vi "Process_Meas_Data.vi"(4 "All queue elements?":bool, 6 "Queues":T4, 7 "One Seconds in":T1 {"Slave"."Ch1 High" format="%0.0f"; "Master"."Ch1 High" format="%0.0f"}, 8 "Status/Errors in":refnum<vi>, 10 "Process data parameters in":T5={"Stop loop"={"Settings changed?"=FALSE, "Stop?"=refnum}, "Button refs"={"Stop program"=refnum, "Save settings"=refnum, "DAQ mode"=refnum, "Reset settings"=refnum, "Apply settings"=refnum, "Reset MAS"=refnum, "Reset SLV"=refnum, "Local DBase?"=refnum, "Last value DBase"=FALSE, "Database"=refnum, "Calibration"=refnum, "Save settings 2"=refnum}, "Process messages"={"Process message mode"=enum."Error", "Slave data?"=FALSE, "Length get settings message"=0, "Delta time"=0.0, "Data_Filter"={"Filter_Data"=FALSE, "Use_Thresh"=FALSE, "Reduce data?"=FALSE}, "Time_difference_stack"=[], "Starting sec"=0, "Ending sec"=0, "Ending sec 2"=0, "MAS_Page_Thresh"=refnum, "SLV_Page_Thresh"=refnum, "Database"=refnum}, "Settings state"={"MAS locked?"=refnum, "SLV locked?"=refnum}, "Mode"={"Mode"=enum."Dialog", "Expert?"=FALSE, "Dialog?"=FALSE}, "Alignment parameters"=refnum, "Timer parameters"=refnum, "Files"={"Path config file"=path "", "Path def. ini file"=path "", "Path ini file 1"=path "", "Path ini file 2"=path "", "Path RBF file"=path ""}, "Time difference"=refnum, "Alignment"={"GEN_Page_Calibrate"=refnum, "MAS_Page_Gain"=refnum, "MAS_Page_Offset"=refnum, "SLV_Page_Gain"=refnum, "SLV_Page_Offset"=refnum, "MAS_Page_Common"=refnum, "SLV_Page_Common"=refnum}, "Page Statistics"=refnum}, 11 "Devices in":T14) -> (0 "Status/Errors out":refnum<vi>, 2 "Process data parameters out":T5={"Stop loop"={"Settings changed?"=FALSE, "Stop?"=refnum}, "Button refs"={"Stop program"=refnum, "Save settings"=refnum, "DAQ mode"=refnum, "Reset settings"=refnum, "Apply settings"=refnum, "Reset MAS"=refnum, "Reset SLV"=refnum, "Local DBase?"=refnum, "Last value DBase"=FALSE, "Database"=refnum, "Calibration"=refnum, "Save settings 2"=refnum}, "Process messages"={"Process message mode"=enum."Error", "Slave data?"=FALSE, "Length get settings message"=0, "Delta time"=0.0, "Data_Filter"={"Filter_Data"=FALSE, "Use_Thresh"=FALSE, "Reduce data?"=FALSE}, "Time_difference_stack"=[], "Starting sec"=0, "Ending sec"=0, "Ending sec 2"=0, "MAS_Page_Thresh"=refnum, "SLV_Page_Thresh"=refnum, "Database"=refnum}, "Settings state"={"MAS locked?"=refnum, "SLV locked?"=refnum}, "Mode"={"Mode"=enum."Dialog", "Expert?"=FALSE, "Dialog?"=FALSE}, "Alignment parameters"=refnum, "Timer parameters"=refnum, "Files"={"Path config file"=path "", "Path def. ini file"=path "", "Path ini file 1"=path "", "Path ini file 2"=path "", "Path RBF file"=path ""}, "Time difference"=refnum, "Alignment"={"GEN_Page_Calibrate"=refnum, "MAS_Page_Gain"=refnum, "MAS_Page_Offset"=refnum, "SLV_Page_Gain"=refnum, "SLV_Page_Offset"=refnum, "MAS_Page_Common"=refnum, "SLV_Page_Common"=refnum}, "Page Statistics"=refnum}, 3 "Devices out":T14, 5 "One Seconds out":T1 {"Slave"."Ch1 High" format="%0.0f"; "Master"."Ch1 High" format="%0.0f"})   [LabVIEW 2013]
uses:
  Controls/Devices.ctl
  Controls/Process_Data_Parameters.ctl
  Controls/Stop_Loop.ctl
  Controls/Button_Refs.ctl
  Controls/Process_Messages.ctl
  Controls/Process_Message_Mode.ctl
  Controls/Settings_State.ctl
  Controls/Mode.ctl
  Controls/Files.ctl
  Controls/Page_Calibration.ctl
  Controls/Queues.ctl
  Controls/One_Second.ctl
  Controls/GPS_Timestamp.ctl
  Controls/One_Seconds.ctl
  Controls/Found_SLV_Data.ctl
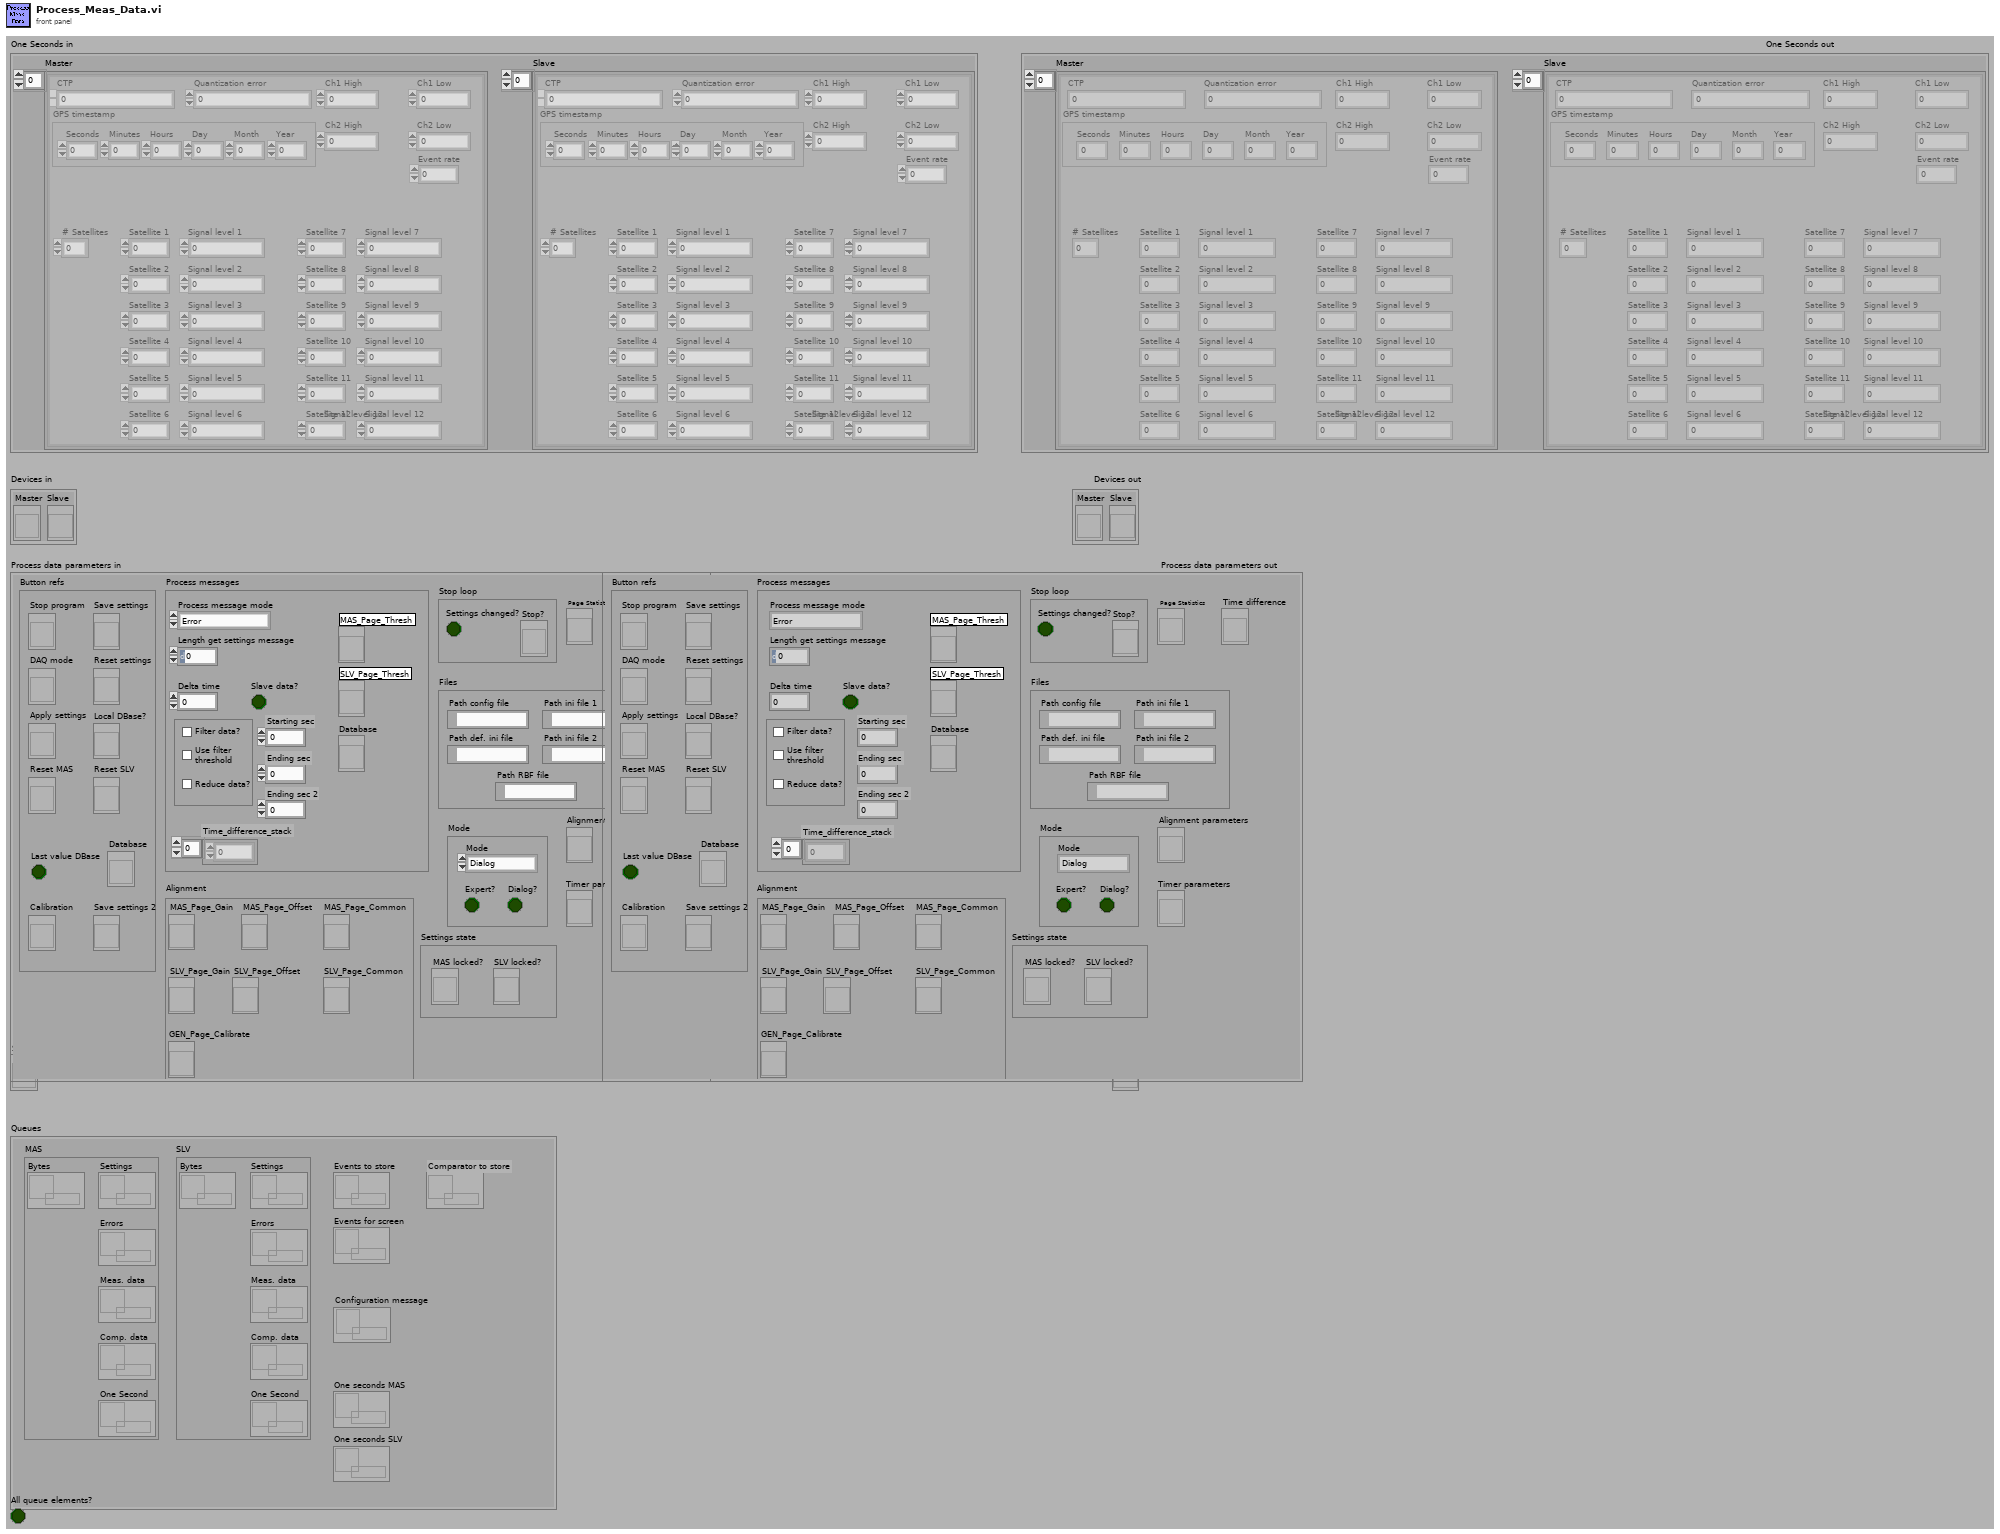
[diagram p1: front panel]
types:
  T1 = typedef "One_Seconds.ctl" = cluster{"Master":T2[], "Slave":T2[]}
  T2 = typedef "One_Second.ctl" = cluster{"GPS timestamp":T3, "CTP":u32, "Quantization error":u32, "Ch1 High":u16, "Ch1 Low":u16, "Ch2 High":u16, "Ch2 Low":u16, "Event rate":u16, "# Satellites":u8, "Satellite 1":u8, "Satellite 2":u8, "Satellite 3":u8, "Satellite 4":u8, "Satellite 5":u8, "Satellite 6":u8, "Signal level 1":sgl, "Signal level 2":sgl, "Signal level 3":sgl, "Signal level 4":sgl, "Signal level 5":sgl, "Signal level 6":sgl, "Satellite 7":u8, "Satellite 8":u8, "Satellite 9":u8, "Satellite 10":u8, "Satellite 11":u8, "Satellite 12":u8, "Signal level 7":sgl, "Signal level 8":sgl, "Signal level 9":sgl, "Signal level 10":sgl, "Signal level 11":sgl, "Signal level 12":sgl}
  T3 = typedef "GPS_Timestamp.ctl" = cluster{"Seconds":u8, "Minutes":u8, "Hours":u8, "Day":u8, "Month":u8, "Year":u16}
  T4 = typedef "Queues.ctl" = cluster{"MAS":cluster{"Bytes":refnum<queue>, "Settings":refnum<queue>, "Errors":refnum<queue>, "Meas. data":refnum<queue>, "One Second":refnum<queue>, "Comp. data":refnum<queue>}, "SLV":cluster{"Bytes":refnum<queue>, "Settings":refnum<queue>, "Errors":refnum<queue>, "Meas. data":refnum<queue>, "One Second":refnum<queue>, "Comp. data":refnum<queue>}, "Events to store":refnum<queue>, "Events for screen":refnum<queue>, "One seconds MAS":refnum<queue>, "One seconds SLV":refnum<queue>, "Configuration message":refnum<queue>, "Comparator to store":refnum<queue>}
  T5 = typedef "Process_Data_Parameters.ctl" = cluster{"Stop loop":T6, "Button refs":T7, "Process messages":T8, "Settings state":T10, "Mode":T11, "Alignment parameters":refnum<vi>, "Timer parameters":refnum<vi>, "Files":T12, "Time difference":refnum<vi>, "Alignment":T13, "Page Statistics":refnum<vi>}
  T6 = typedef "Stop_Loop.ctl" = cluster{"Settings changed?":bool, "Stop?":refnum<vi>}
  T7 = typedef "Button_Refs.ctl" = cluster{"Stop program":refnum<vi>, "Save settings":refnum<vi>, "DAQ mode":refnum<vi>, "Reset settings":refnum<vi>, "Apply settings":refnum<vi>, "Reset MAS":refnum<vi>, "Reset SLV":refnum<vi>, "Local DBase?":refnum<vi>, "Last value DBase":bool, "Database":refnum<vi>, "Calibration":refnum<vi>, "Save settings 2":refnum<vi>}
  T8 = typedef "Process_Messages.ctl" = cluster{"Process message mode":T9, "Slave data?":bool, "Length get settings message":i32, "Delta time":dbl, "Data_Filter":cluster{"Filter_Data":bool, "Use_Thresh":bool, "Reduce data?":bool}, "Time_difference_stack":u64[], "Starting sec":u64, "Ending sec":u64, "Ending sec 2":u64, "MAS_Page_Thresh":refnum<vi>, "SLV_Page_Thresh":refnum<vi>, "Database":refnum<vi>}
  T9 = typedef "Process_Message_Mode.ctl" = enum16{"Error", "Measurement data", "Comparator data", "One Second"}
  T10 = typedef "Settings_State.ctl" = cluster{"MAS locked?":refnum<vi>, "SLV locked?":refnum<vi>}
  T11 = typedef "Mode.ctl" = cluster{"Mode":enum8{"Stop", "Dialog", "Hisparc II", "Hisparc II DAQ", "Alignment"}, "Expert?":bool, "Dialog?":bool}
  T12 = typedef "Files.ctl" = cluster{"Path config file":path, "Path def. ini file":path, "Path ini file 1":path, "Path ini file 2":path, "Path RBF file":path}
  T13 = typedef "Page_Calibration.ctl" = cluster{"GEN_Page_Calibrate":refnum<vi>, "MAS_Page_Gain":refnum<vi>, "MAS_Page_Offset":refnum<vi>, "SLV_Page_Gain":refnum<vi>, "SLV_Page_Offset":refnum<vi>, "MAS_Page_Common":refnum<vi>, "SLV_Page_Common":refnum<vi>}
  T14 = typedef "Devices.ctl" = cluster{"Master":refnum<vi>, "Slave":refnum<vi>}
  T15 = enum8{"Stop", "Dialog", "Hisparc II", "Hisparc II DAQ", "Alignment"}
  T16 = typedef "Found_SLV_Data.ctl" = cluster{"Found SLV data?":bool, "Wait for SLV data?":bool}
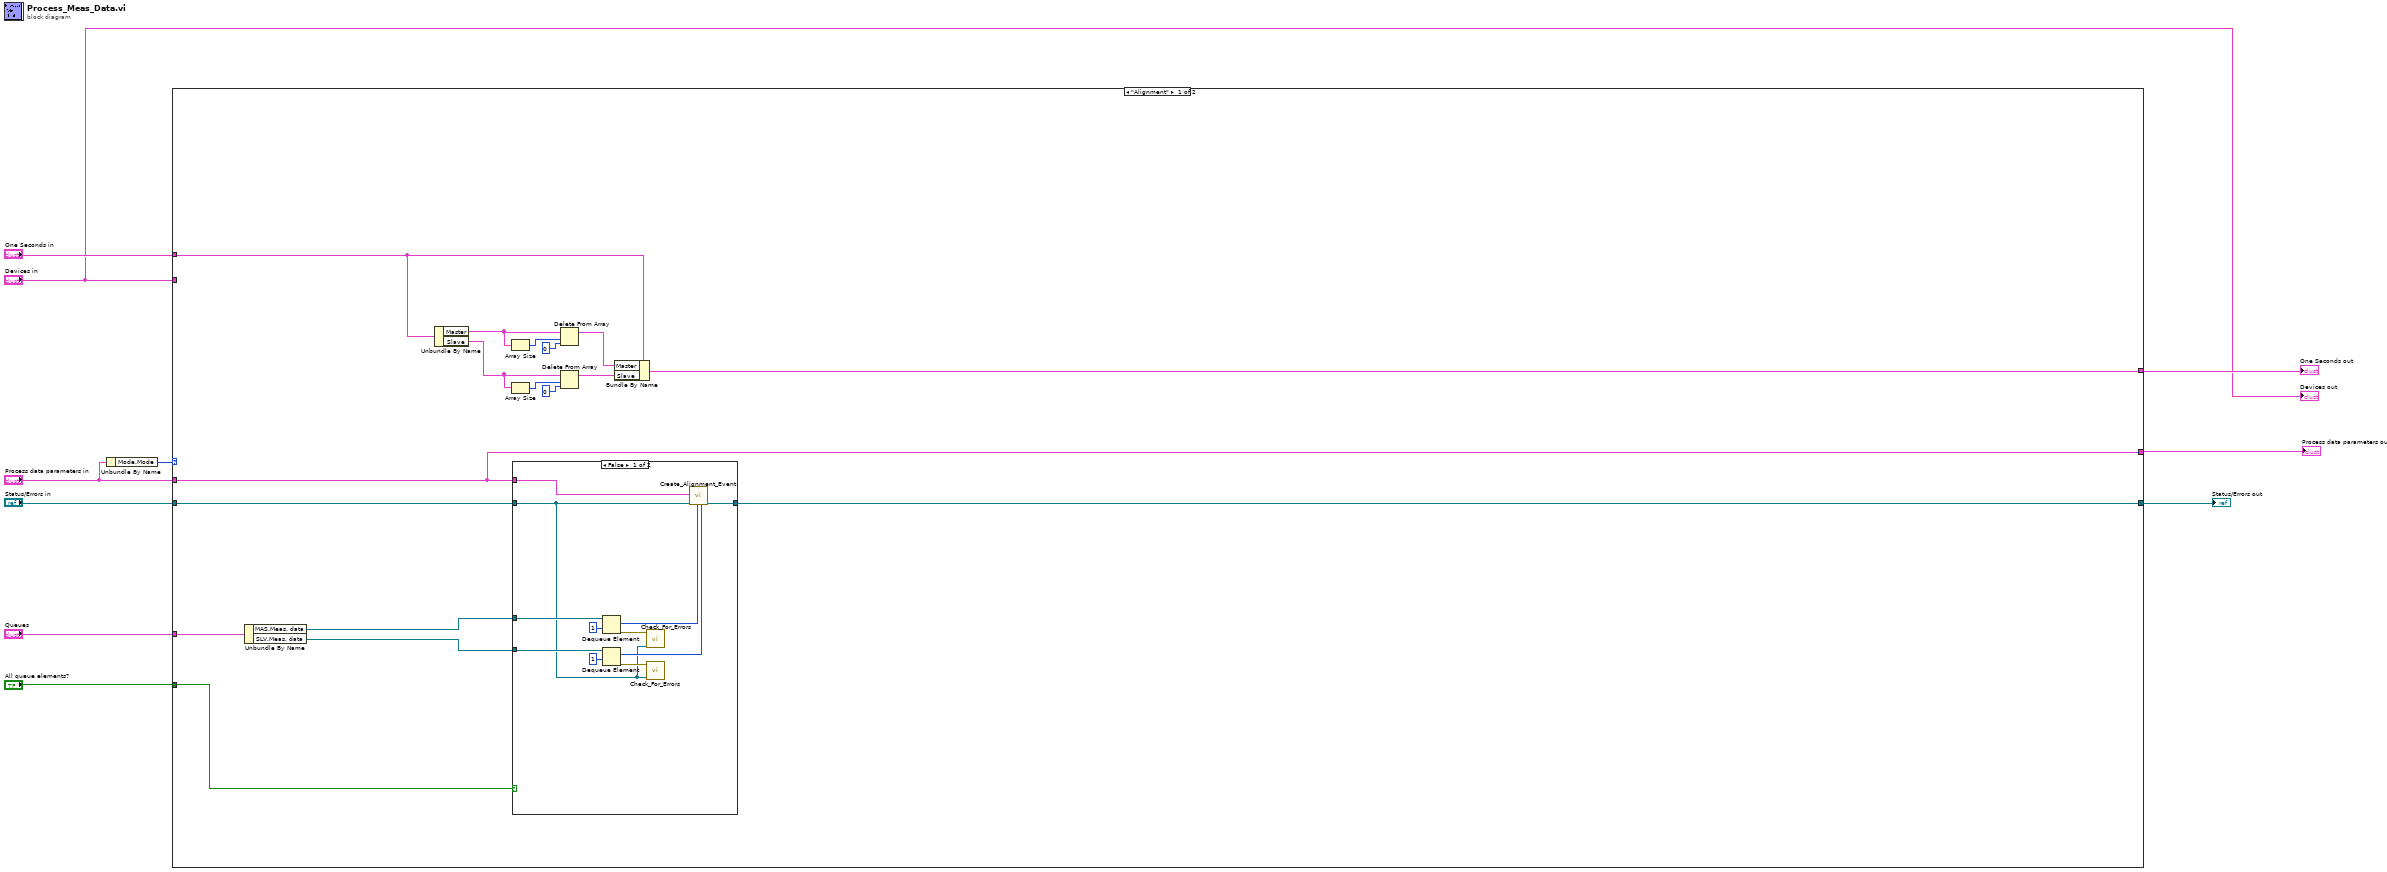
[diagram p0: block diagram]
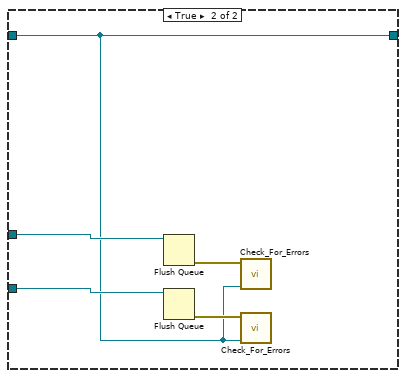
[diagram p2: hidden frame]
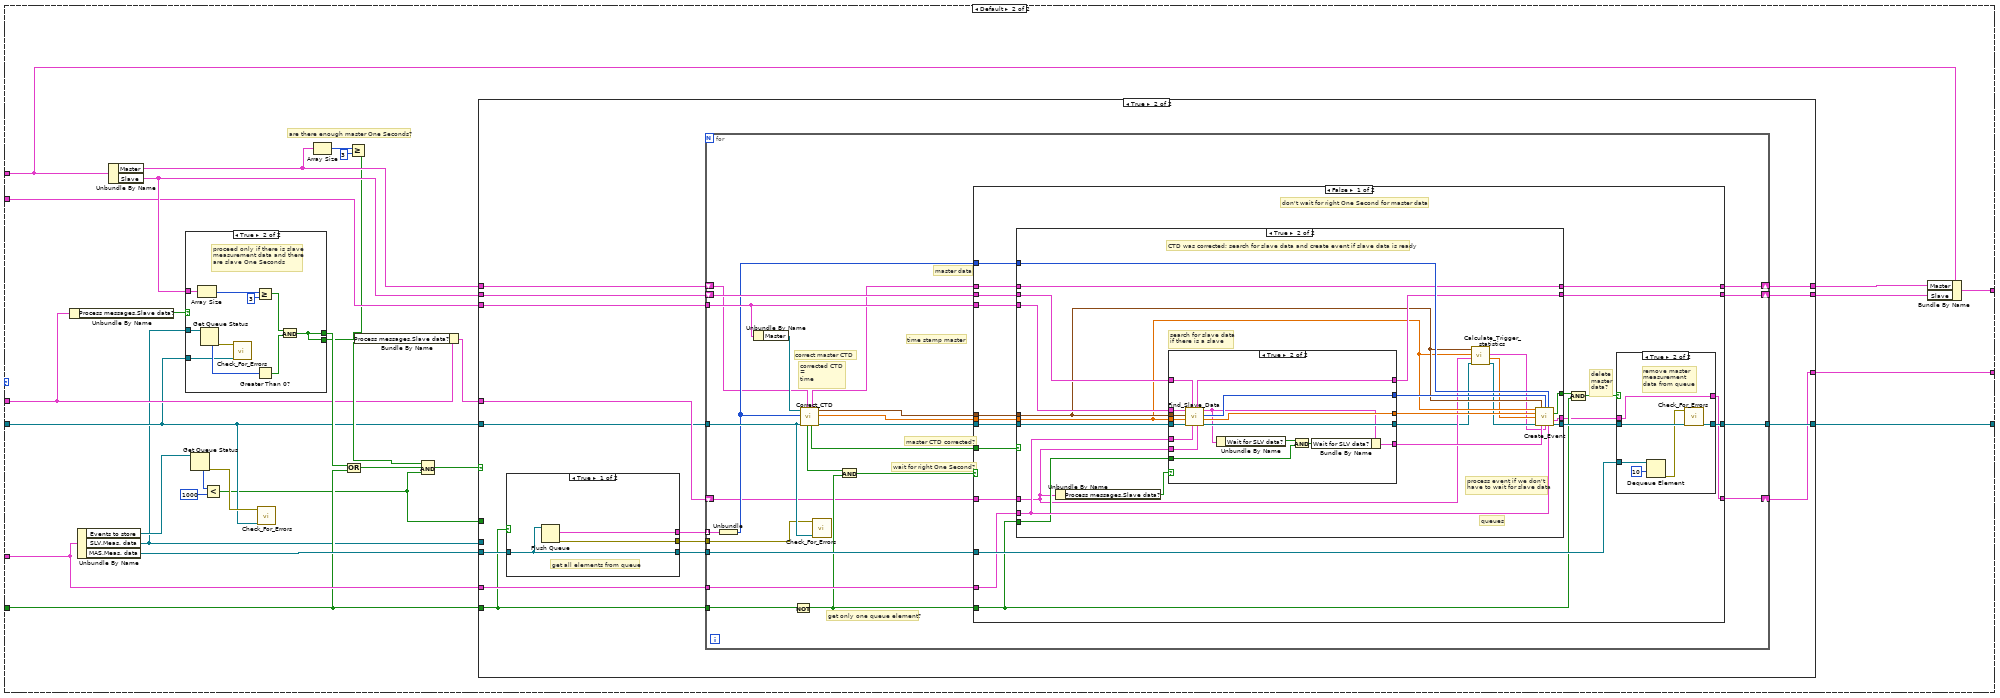
[diagram p3: hidden frame]
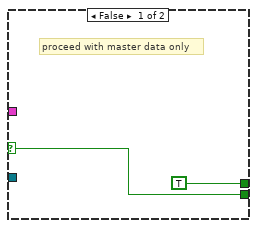
[diagram p4: hidden frame]
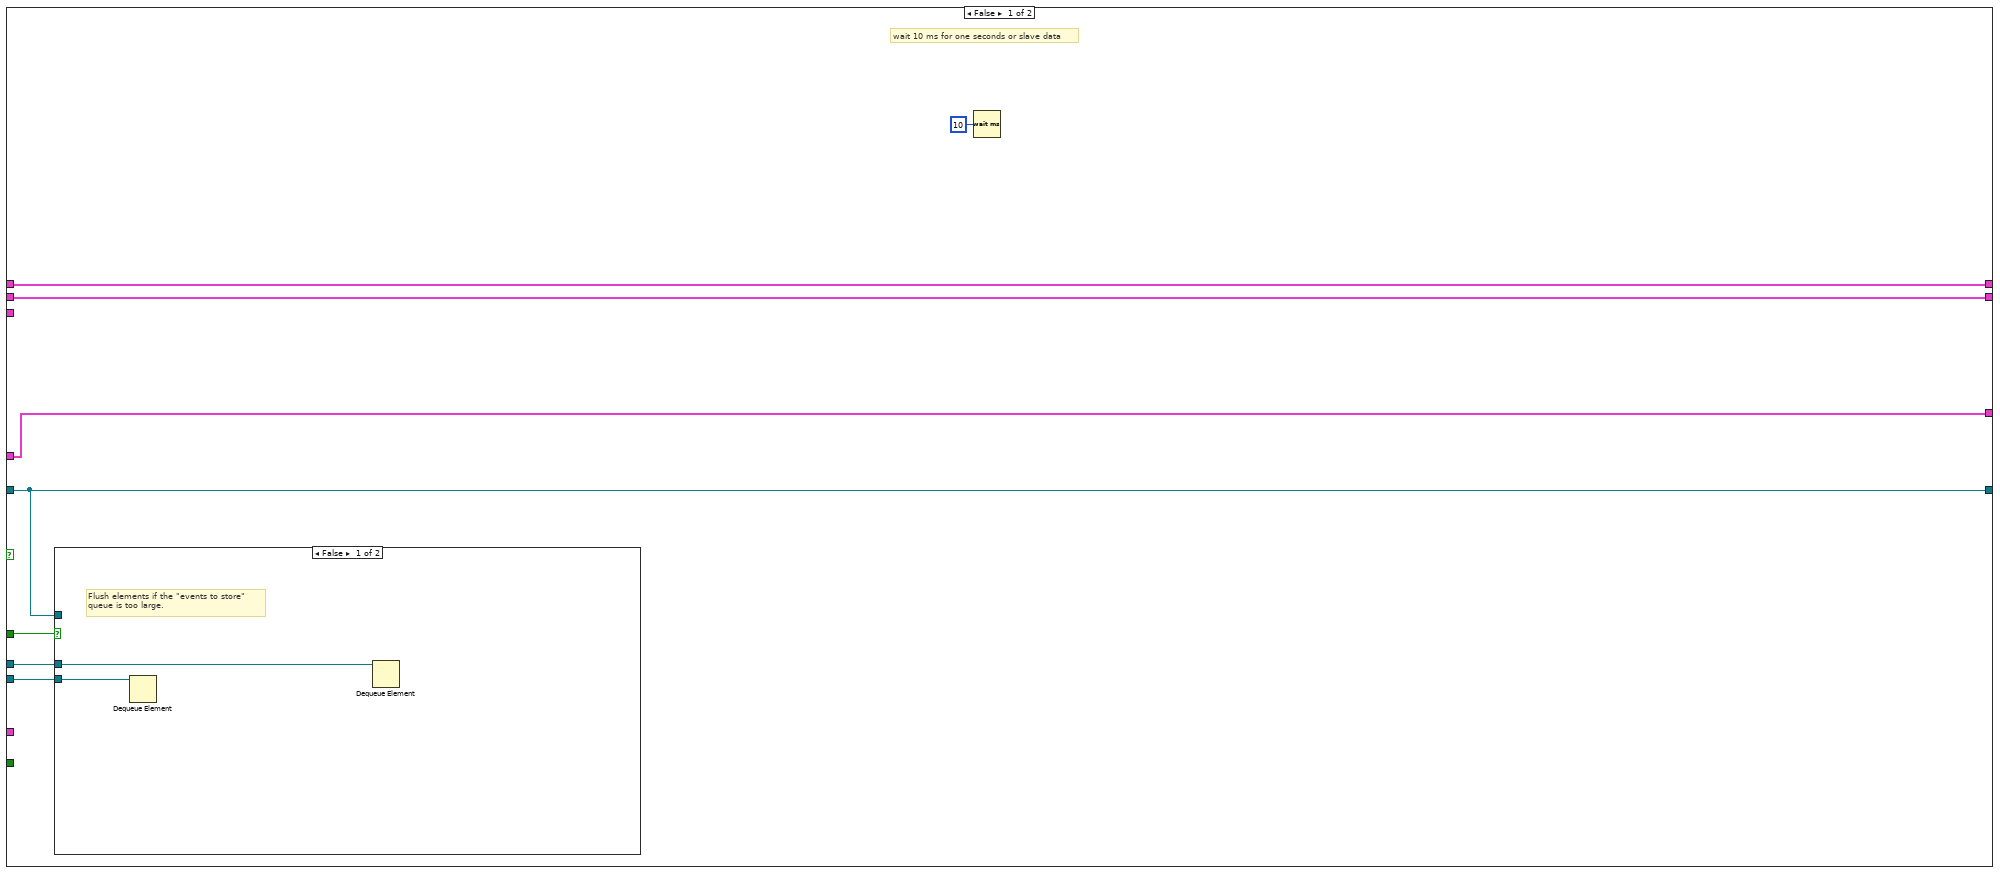
[diagram p5: hidden frame]
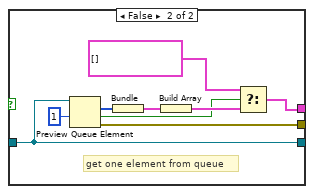
[diagram p7: hidden frame]
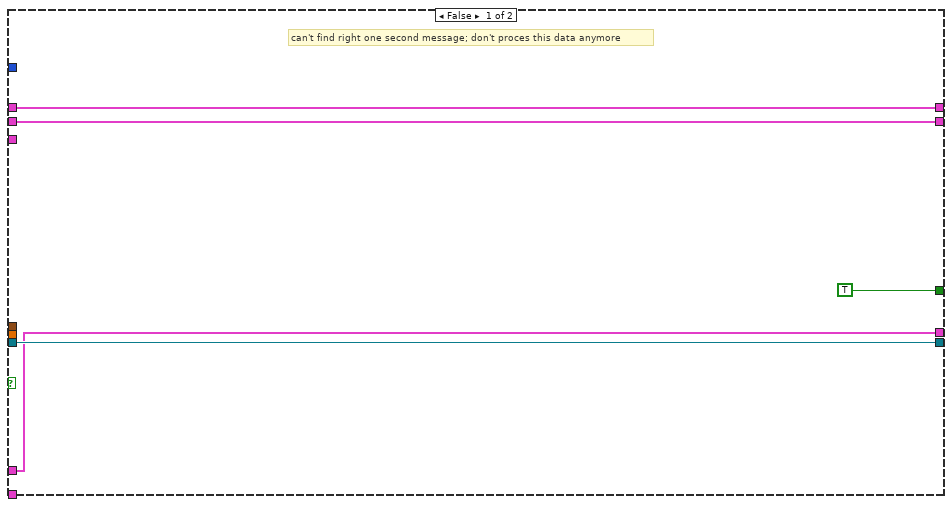
[diagram p9: hidden frame]
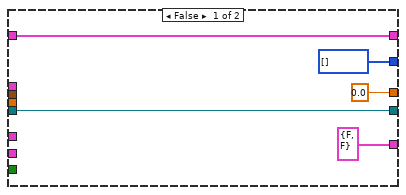
[diagram p10: hidden frame]
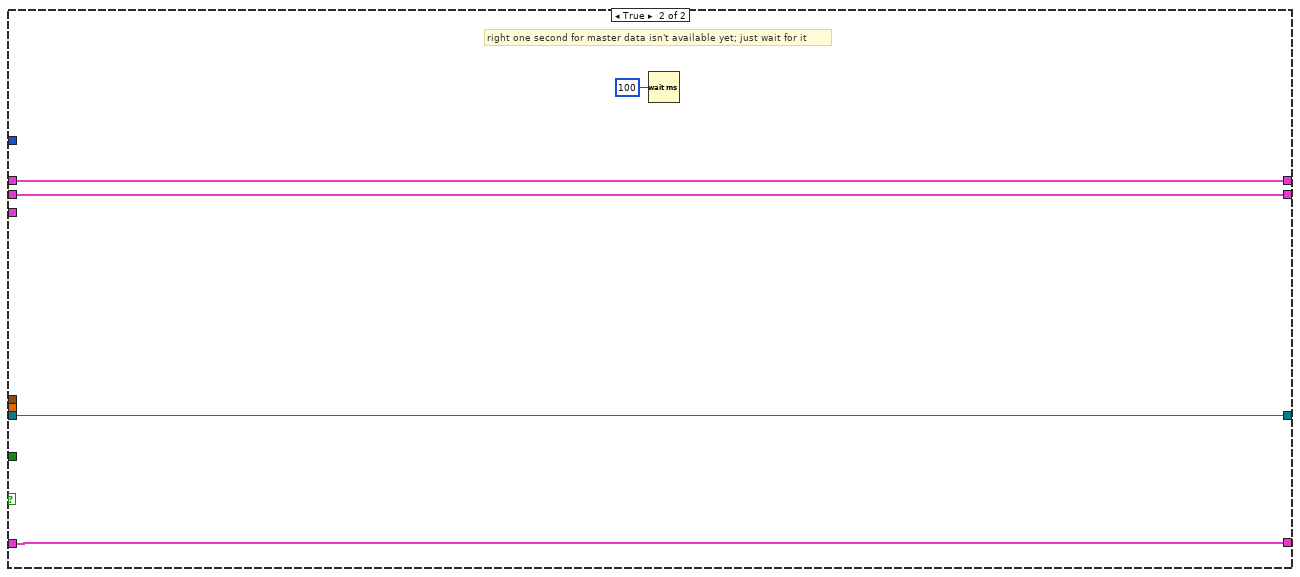
[diagram p11: hidden frame]
diagram:
  n1 = Unbundle By Name("Process data parameters in") -> ("Mode.Mode"=w5:T15)
  n2 = case shown="\"Alignment\"" w5 {
    tunnel: [w22 w72] -> w3
    tunnel: [w12 w68] -> w10
    tunnel: "One Seconds in" -> [w13 w67]
    tunnel: "Queues" -> [w27 w65]
    tunnel: "All queue elements?" -> [w26 w61]
    tunnel: "Devices in" -> [_ w59]
    tunnel: "Status/Errors in" -> [w25 w47]
    tunnel: "Process data parameters in" -> [w11 w52]
    tunnel: [w11 w44] -> w1
    frame "Alignment" {
      n3 = Unbundle By Name(w27) -> ("MAS.Meas. data"=w24:refnum<queue>, "SLV.Meas. data"=w23:refnum<queue>)
      n4 = Unbundle By Name(w13) -> ("Master"=w21:T2[], "Slave"=w16:T2[])
      n5 = Array Size(array=w21) -> (size(s)=w20:i32)
      n6 = Array Size(array=w16) -> (size(s)=w18:i32)
      n7 = case shown="False" w26 {
        tunnel: w25 -> [w30 w39]
        tunnel: w24 -> [w38 w41]
        tunnel: w23 -> [w35 w40]
        tunnel: w11 -> [w29 _]
        tunnel: [w28 w39] -> w22
        frame False {
          n8 = Dequeue Element(queue=w38, timeout in ms (-1)=1) -> (element=w34:u8[], error out=w32:errorcluster)  [unwired: 1 in, 2 out]
          n9 = Dequeue Element(queue=w35, timeout in ms (-1)=1) -> (element=w33:u8[], error out=w31:errorcluster)  [unwired: 1 in, 2 out]
          n10 = call "Check_For_Errors.vi"("Status/Errors in"=w30, "error in"=w32) -> ()  [unwired: 10 out]
          n11 = call "Check_For_Errors.vi"("Status/Errors in"=w30, "error in"=w31) -> ()  [unwired: 10 out]
          n12 = call "Create_Alignment_Event.vi"("Slave data"=w33, "Master data"=w34, "Status/Errors in"=w30, "Process data parameters in"=w29) -> ("Status/Errors out"=w28:refnum<vi>)  [unwired: 2 in, 5 out]
        }
        frame True {
          n13 = Flush Queue(queue=w41) -> (error out=w43:errorcluster)  [unwired: 1 in, 2 out]
          n14 = Flush Queue(queue=w40) -> (error out=w42:errorcluster)  [unwired: 1 in, 2 out]
          n15 = call "Check_For_Errors.vi"("Status/Errors in"=w39, "error in"=w43) -> ()  [unwired: 10 out]
          n16 = call "Check_For_Errors.vi"("Status/Errors in"=w39, "error in"=w42) -> ()  [unwired: 10 out]
        }
      }
      n17 = Delete From Array(array=w21, length=w20, index=0) -> (array with subset deleted=w15:T2[])  [unwired: 1 out]
      n18 = Delete From Array(array=w16, length=w18, index=0) -> (array with subset deleted=w14:T2[])  [unwired: 1 out]
      n19 = Bundle By Name(cluster=w13, "Master"=w15, "Slave"=w14) -> (w12:T1)
    }
    frame Default {
      # "are there enough master One Seconds?"
      n20 = Unbundle By Name(w52) -> ("Process messages.Slave data?"=w71:bool)
      n21 = Unbundle By Name(w65) -> ("Events to store"=w51:refnum<queue>, "SLV.Meas. data"=w46:refnum<queue>, "MAS.Meas. data"=w66:refnum<queue>)
      n22 = Unbundle By Name(w67) -> ("Master"=w56:T2[], "Slave"=w60:T2[])
      n23 = case shown="True" w71 {
        selector: w71 -> [w73 _]
        tunnel: [TRUE w77] -> w63
        tunnel: w46 -> [_ w82]
        tunnel: w47 -> [_ w81]
        tunnel: w60 -> [_ w80]
        tunnel: [w73 w77] -> w62
        frame False {
          # "proceed with master data only"
        }
        frame True {
          # "proceed only if there is slave\nmeasurement data and there\nare slave One Seconds"
          n24 = Array Size(array=w80) -> (size(s)=w76:i32)
          n25 = Get Queue Status(queue=w82) -> (error out=w83:errorcluster, # elements in queue=w84:i32)  [unwired: 1 in, 7 out]
          n26 = call "Check_For_Errors.vi"("Status/Errors in"=w81, "error in"=w83) -> ()  [unwired: 10 out]
          n27 = Greater Or Equal?(x=w76, y=3) -> (x >= y?=w78:bool)
          n28 = Greater Than 0?(x=w84) -> (x > 0?=w79:bool)
          n29 = And(x=w78, y=w79) -> (x .and. y?=w77:bool)
        }
      }
      n30 = Get Queue Status(queue=w51) -> (error out=w48:errorcluster, # elements in queue=w49:i32)  [unwired: 1 in, 7 out]
      n31 = Less?(x=w49, y=1000) -> (x < y?=w45:bool)
      n32 = call "Check_For_Errors.vi"("Status/Errors in"=w47, "error in"=w48) -> ()  [unwired: 10 out]
      n33 = Array Size(array=w56) -> (size(s)=w58:i32)
      n34 = Or(x=w63, y=w61) -> (x .or. y?=w54:bool)
      n35 = Greater Or Equal?(x=w58, y=3) -> (x >= y?=w53:bool)
      n36 = Bundle By Name(cluster=w52, "Process messages.Slave data?"=w62) -> (w64:T5)
      n37 = Compound Arithmetic op=AND(w53, w54, w45) -> (w55:bool)
      n38 = case shown="True" w55 {
        tunnel: [w87 w109] -> w72
        tunnel: w64 -> [w85 w108]
        tunnel: w47 -> [w87 w107]
        tunnel: w66 -> [w89 w105]
        tunnel: w59 -> [_ w104]
        tunnel: w56 -> [w90 w100]
        tunnel: [w90 w103] -> w70
        tunnel: w60 -> [w91 w102]
        tunnel: [w91 w99] -> w69
        tunnel: w65 -> [_ w101]
        tunnel: w61 -> [_ w96]
        tunnel: w46 -> [w88 _]
        tunnel: w45 -> [w86 _]
        tunnel: [w85 w95] -> w44
        frame False {
          # "wait 10 ms for one seconds or slave data"
          n39 = case shown="False" w86 {
            tunnel: w89 -> [w94 _]
            tunnel: w88 -> [w93 _]
            tunnel: w87 -> [_ _]
            frame False {
              # "Flush elements if the \"events to store\" \nqueue is too large."
              n40 = Dequeue Element(queue=w94) -> ()  [unwired: 1 in, 5 out]
              n41 = Dequeue Element(queue=w93) -> ()  [unwired: 1 in, 5 out]
            }
            frame True {
            }
          }
          n42 = Wait (ms)(milliseconds to wait=u32 10) -> ()  [unwired: 1 out]
        }
        frame True {
          n43 = case shown="True" w96 {
            tunnel: [w112 w121] -> w106
            tunnel: w105 -> [w110 w118]
            tunnel: [w111 w114] -> w98
            tunnel: [w110 w118] -> w97
            frame True {
              # "get all elements from queue"
              n44 = Flush Queue(queue=w110) -> (remaining elements=w111:cluster{u8[]}[], error out=w112:errorcluster)  [unwired: 1 in, 1 out]
            }
            frame False {
              # "get one element from queue"
              n45 = Preview Queue Element(queue=w118, timeout in ms (-1)=1) -> (element=w120:u8[], timed out?=w115:bool, error out=w121:errorcluster)  [unwired: 1 in, 1 out]
              n46 = Bundle(w120) -> (w119:cluster{u8[]})  [unwired: 1 in]
              n47 = Build Array(w119) -> (w116:cluster{u8[]}[])
              n48 = Select(t=cluster{u8[]}[] [], s=w115, f=w116) -> (s? t:f=w114:cluster{u8[]}[])
            }
          }
          n49 = for {
            tunnel: [w144] -> w109
            tunnel: w107 -> [w143]
            tunnel: w106 -> [w142]
            tunnel: w97 -> [w141]
            tunnel: w98 -> [w140] mode=indexing
            tunnel: w104 -> [w139]
            tunnel: w101 -> [w138]
            shift-right: [w126] -> w103
            shift-left: w100 -> [w131]
            shift-right: [w136] -> w99
            shift-left: w102 -> [w137]
            tunnel: w96 -> [w134]
            shift-right: [w128] -> w95
            shift-left: w108 -> [w122]
            # "get only one queue element?"
            # "time stamp master"
            # "corrected CTD\n=\ntime"
            # "master data"
            # "correct master CTD"
            # "master CTD corrected?"
            # "wait for right One Second?"
            n50 = Unbundle(w140) -> (w135:u8[])
            n51 = Unbundle By Name(w139) -> ("Master"=w145:refnum<vi>)
            n52 = Not(x=w134) -> (.not. x?=w132:bool)
            n53 = call "Correct_CTD.vi"("One Second in"=w131, "Status/Errors in"=w143, "Message in"=w135, "Device in"=w145) -> ("Status/Errors out"=w123:refnum<vi>, "Time"=w125:dbl, "GPS timestamp out"=w124:T3, "CTD corrected?"=w129:bool, "One Second out"=w127:T2[], "Wait for tick count?"=w130:bool)  [unwired: 2 out]
            n54 = call "Check_For_Errors.vi"("Status/Errors in"=w143, "error in"=w142) -> ()  [unwired: 10 out]
            n55 = And(x=w130, y=w132) -> (x .and. y?=w133:bool)
            n56 = case shown="False" w133 {
              tunnel: [w156 w226] -> w144
              tunnel: w123 -> [w165 w226]
              tunnel: w139 -> [w164 _]
              tunnel: w129 -> [w162 _]
              tunnel: w141 -> [w163 _]
              tunnel: w122 -> [w158 w223]
              tunnel: w124 -> [w160 _]
              tunnel: w125 -> [w159 _]
              tunnel: w135 -> [w161 _]
              tunnel: w137 -> [w155 w224]
              tunnel: [w154 w224] -> w136
              tunnel: w138 -> [w153 _]
              tunnel: w132 -> [w150 _]
              tunnel: [w148 w223] -> w128
              tunnel: w127 -> [w147 w222]
              tunnel: [w146 w222] -> w126
              frame False {
                # "delete\nmaster\ndata?"
                # "don't wait for right One Second for master data"
                n57 = case shown="True" w162 {
                  tunnel: w164 -> [_ w199]
                  tunnel: [w178 w190] -> w157
                  tunnel: w165 -> [w178 w200]
                  tunnel: w160 -> [_ w185]
                  tunnel: w159 -> [_ w184]
                  tunnel: [TRUE w192] -> w151
                  tunnel: w161 -> [_ w196]
                  tunnel: w158 -> [w175 w183]
                  tunnel: w155 -> [w176 w197]
                  tunnel: [w176 w187] -> w154
                  tunnel: w153 -> [_ w193]
                  tunnel: w150 -> [_ w191]
                  tunnel: [w175 w188] -> w149
                  tunnel: w147 -> [w174 w186]
                  tunnel: [w174 w186] -> w146
                  frame False {
                    # "can't find right one second message; don't proces this data anymore"
                  }
                  frame True {
                    # "search for slave data\nif there is a slave"
                    # "process event if we don't\nhave to wait for slave data"
                    # "queues"
                    # "CTD was corrected; search for slave data and create event if slave data is ready"
                    n58 = Unbundle By Name(w183) -> ("Process messages.Slave data?"=w198:bool)
                    n59 = case shown="True" w198 {
                      tunnel: w200 -> [w205 w213]
                      tunnel: [w205 w211] -> w182
                      tunnel: w199 -> [_ w221]
                      tunnel: w185 -> [_ w220]
                      tunnel: w184 -> [_ w219]
                      tunnel: [u8[] [] ("Slave data") w218] -> w195
                      tunnel: [0.0 ("CTDM slave") w217] -> w194
                      tunnel: w197 -> [w202 w216]
                      tunnel: [w202 w215] -> w187
                      tunnel: w193 -> [_ w214]
                      tunnel: w183 -> [_ w212]
                      tunnel: [T16 {"Found SLV data?"=FALSE, "Wait for SLV data?"=FALSE} ("Found SLV data?") w206] -> w189
                      tunnel: w191 -> [_ w209]
                      frame False {
                      }
                      frame True {
                        n60 = call "Find_Slave_Data.vi"("Process data parameters in"=w212, "Queues"=w214, "One Second in"=w216, "Status/Errors in"=w213, "Time master"=w219, "GPS timestamp master"=w220, "Devices"=w221) -> ("Status/Errors out"=w211:refnum<vi>, "Time delta slave"=w217:dbl, "Slave data"=w218:u8[], "Found SLV data?"=w208:T16, "One Second out"=w215:T2[])
                        n61 = Unbundle By Name(w208) -> ("Wait for SLV data?"=w210:bool)
                        n62 = And(x=w210, y=w209) -> (x .and. y?=w207:bool)
                        n63 = Bundle By Name(cluster=w208, "Wait for SLV data?"=w207) -> (w206:T16)
                      }
                    }
                    n64 = call "Calculate_Trigger_statistics.vi"("Status/Errors in"=w182, "Process data parameters in"=w183, "Time"=w184, "GPS timestamp in"=w185) -> ("Status/Errors out"=w181:refnum<vi>, "Trigger rate /s"=w180:dbl, "Process data parameters out"=w179:T5)  [unwired: 5 out]
                    n65 = call "Create_Event.vi"("Time master"=w184, "GPS timestamp master"=w185, "Slave data"=w195, "Master data"=w196, "Time delta slave"=w194, "Trigger rate /m"=w180, "Status/Errors in"=w181, "Found SLV data?"=w189, "Process data parameters in"=w179, "Queues"=w193) -> ("Delete master data?"=w192:bool, "Process data parameters out"=w188:T5, "Status/Errors out"=w190:refnum<vi>)  [unwired: 3 out]
                  }
                }
                n66 = And(x=w151, y=w150) -> (x .and. y?=w152:bool)
                n67 = case shown="True" w152 {
                  tunnel: w163 -> [_ w173]
                  tunnel: w157 -> [w167 w172]
                  tunnel: [w167 w170] -> w156
                  tunnel: w149 -> [w166 w168]
                  tunnel: [w166 w168] -> w148
                  frame False {
                    # "keep master measurement\ndata in queue for now"
                  }
                  frame True {
                    # "remove master\nmeasurement\ndata from queue"
                    n68 = Dequeue Element(queue=w173, timeout in ms (-1)=10) -> (error out=w171:errorcluster)  [unwired: 1 in, 3 out]
                    n69 = call "Check_For_Errors.vi"("Status/Errors in"=w172, "error in"=w171) -> ("Status/Errors out"=w170:refnum<vi>)  [unwired: 9 out]
                  }
                }
              }
              frame True {
                # "right one second for master data isn't available yet; just wait for it"
                n70 = Wait (ms)(milliseconds to wait=u32 100) -> ()  [unwired: 1 out]
              }
            }
          }
        }
      }
      n71 = Bundle By Name(cluster=w67, "Master"=w70, "Slave"=w69) -> (w68:T1)
    }
  }
  "Status/Errors out" <- w3
  "Process data parameters out" <- w1
  "One Seconds out" <- w10
  "Devices out" <- "Devices in"
